vi "Sort Selectors.vi"(10 "Unsorted Selectors":string[](array[string])) -> (2 "Sorted Selectors":string[](array[string]))   [LabVIEW 2019, in "LSS.lvlib"]
doc: "Sorts selectors such that they go from least specific to most specific.\n\n<b>Inputs:</b>\n<b>Unsorted Selectors</b> - List of selectors which could potentially be out of order.\n\n<b>Outputs:</b>\n<b>Sorted Selectors</b> - Selectors sorted with least specific items first, most specific items last."
uses:
  LSS.lvlib
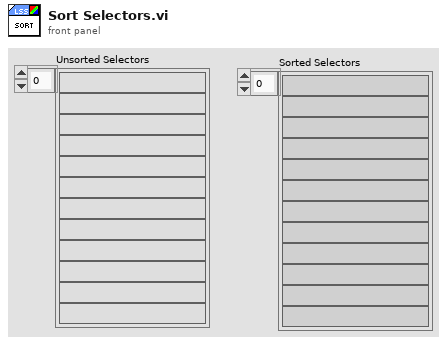
[diagram p1: front panel]
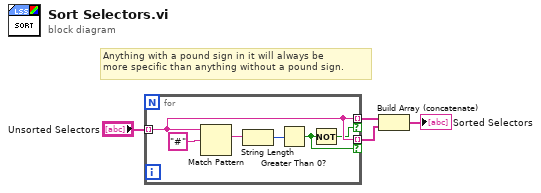
[diagram p0: block diagram]
diagram:
  # "Anything with a pound sign in it will always be\nmore specific than anything without a pound sign."
  n1 = for {
    tunnel: "Unsorted Selectors" -> [w7] mode=indexing
    tunnel: [w7] -> w3 mode=indexing if=w6
    tunnel: [w7] -> w2 mode=indexing if=w5
    n2 = Match Pattern(string=w7, regular expression="#") -> (match substring=w9:string)  [unwired: 1 in, 3 out]
    n3 = String Length(string=w9) -> (length=w8:i32)
    n4 = Greater Than 0?(x=w8) -> (x > 0?=w5:bool)
    n5 = Not(x=w5) -> (.not. x?=w6:bool)
  }
  n6 = Build Array (concatenate)(w3, w2) -> (→"Sorted Selectors":string[])
